vi "Unpack Joysticks.vi"(0 "Ian's Drive":T2, 5 "Ian's Buttons":T1, 11 "Jeffery's Stick":T3) -> (2 "Roller On?":bool, 3 "Ian's shoot?":bool, 4 "Ian up":bool, 6 "Ian down":bool, 8 "Roller speed(raw)":dbl, 10 "Jeffrey down":bool, 14 "Jeffrey shoot?":bool, 15 "Jeffrey up":bool)   [LabVIEW 2013]
uses:
  <vilib>/Rock Robotics/WPI/Joystick/WPI_JoystickDevRef.ctl
  <vilib>/Rock Robotics/WPI/Joystick/WPI_JoystickDeviceEnum.ctl
  <vilib>/Rock Robotics/WPI/Joystick/WPI_JoystickButtonState.ctl
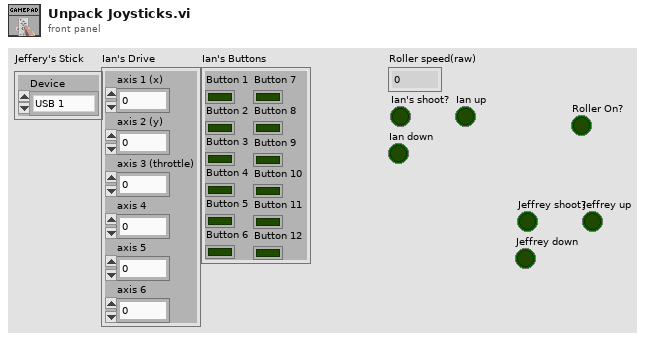
[diagram p1: front panel]
types:
  T1 = typedef "WPI_JoystickButtonState.ctl" = cluster{"Button 1":bool, "Button 2":bool, "Button 3":bool, "Button 4":bool, "Button 5":bool, "Button 6":bool, "Button 7":bool, "Button 8":bool, "Button 9":bool, "Button 10":bool, "Button 11":bool, "Button 12":bool}
  T2 = cluster{"axis 1 (x)":dbl, "axis 2 (y)":dbl, "axis 3 (throttle)":dbl, "axis 4":dbl, "axis 5":dbl, "axis 6":dbl}
  T3 = typedef "WPI_JoystickDevRef.ctl" = cluster{"Device":T4}
  T4 = typedef "WPI_JoystickDeviceEnum.ctl" = enum16{"USB 1", "USB 2", "USB 3", "USB 4", "Kinect 1", "Kinect 2"}
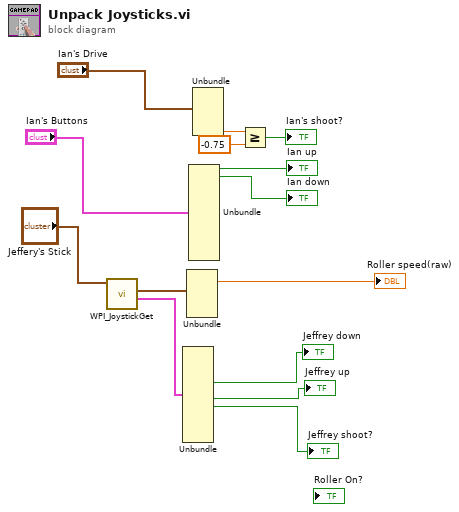
[diagram p0: block diagram]
diagram:
  n1 = call <vilib>:"WPI_JoystickGet.vi"("JoystickDevRef"="Jeffery's Stick") -> ("Buttons"=w14:T1, "Axes"=w13:T2)  [unwired: 4 in, 1 out]
  n2 = Unbundle(w14) -> ("Button 5"=→"Jeffrey down":bool, "Button 7"=→"Jeffrey up":bool, "Button 8"=→"Jeffrey shoot?":bool)  [unwired: 9 out]
  n3 = Unbundle(w13) -> ("axis 2 (y)"=→"Roller speed(raw)":dbl)  [unwired: 5 out]
  n4 = Unbundle("Ian's Buttons") -> ("Button 1"=→"Ian up":bool, "Button 2"=→"Ian down":bool)  [unwired: 10 out]
  n5 = Unbundle("Ian's Drive") -> ("axis 6"=w11:dbl)  [unwired: 5 out]
  n6 = Greater Or Equal?(x=w11, y=-0.75) -> (x >= y?=→"Ian's shoot?":bool)
